vi "FbackCurr_IntToAmmps.vi"(10 "Current Feedback":i16, 11 "Numeric":i32) -> (3 "Measured Current (Amps)":dbl)   [LabVIEW 2011]
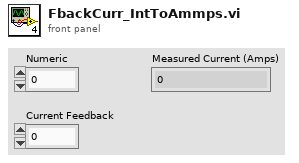
[diagram p1: front panel]
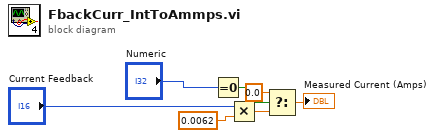
[diagram p0: block diagram]
diagram:
  n1 = Equal To 0?(x="Numeric") -> (x = 0?=w6:bool)
  n2 = Multiply(x="Current Feedback", y=0.0062) -> (x*y=w1:dbl)
  n3 = Select(t=0.0, s=w6, f=w1) -> (s? t:f=→"Measured Current (Amps)":dbl)
